vi "Get_Latest_Experiment_Settings.vi"(8 "error in (no error)":errorcluster) -> (0 "error out":errorcluster, 1 "Experiment":string[](array[string]), 2 "Group":string, 3 "Integer Timestamp":dbl)   [LabVIEW 2013]
uses:
  <vilib>/addons/database/Connection.llb/Conn Execute.vi
  <vilib>/addons/database/Recordset.llb/Rec Fetch Recordset Data (R).vi
  <vilib>/addons/database/Recordset.llb/Rec Destroy - Connection.vi
  <vilib>/addons/database/_DB Variant To Data/Database Variant To Data.xnode
  <vilib>/addons/database/NI_Database_API.lvlib
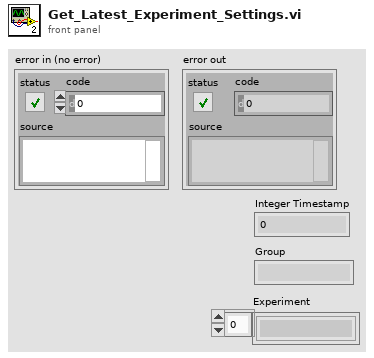
[diagram p1: front panel]
types:
  T1 = typedef "NI_Database_API.lvlib/Conn ObjectReference.ctl" = refnum<k1>
  T2 = typedef "NI_Database_API.lvlib/Rec ObjectReference.ctl" = refnum<k1>
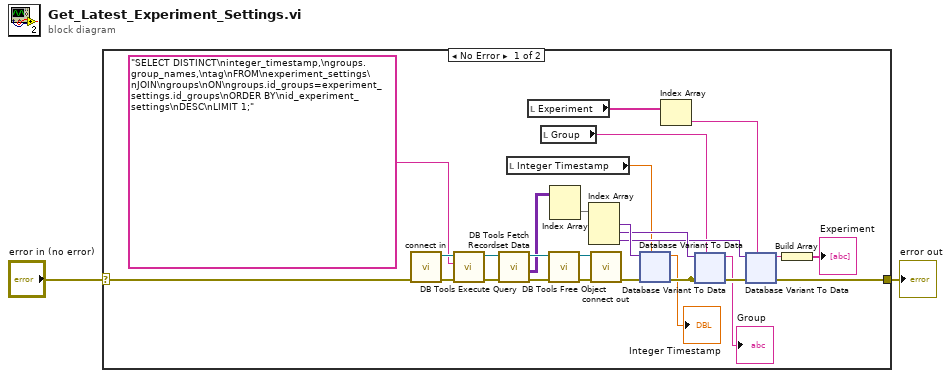
[diagram p0: block diagram]
diagram:
  n1 = case shown="No Error" "error in (no error)" {
    selector: "error in (no error)" -> [w4 w125]
    tunnel: [w16 w125] -> w1
    frame No Error {
      n2 = call "connect in.vi"("error in (no error)"=w4) -> ("error out"=w27:errorcluster, "Database Connection"=w26:T1)  [unwired: 6 in, 1 out]
      n3 = call-poly <vilib>:"DB Tools Execute Query.vi"("error in (no error)"=w27, "SQL query"="SELECT DISTINCT\ninteger_timestamp,\ngroups.group_names,\ntag\nFROM\nexperiment_settings\nJOIN\ngroups\nON\ngroups.id_groups=experiment_settings.id_groups\nORDER BY\nid_experiment_settings\nDESC\nLIMIT 1;" ("format string"), "connection reference"=w26) -> ("error out"=w25:errorcluster, "recordset reference"=w24:T2)  [unwired: 5 in]
      n4 = call-poly <vilib>:"DB Tools Fetch Recordset Data.vi"("error in (no error)"=w25, "recordset reference"=w24) -> ("error out"=w23:errorcluster, "recordset data"=w19:variant[][], "recordset reference out"=w28:T2)  [unwired: 3 in]
      n5 = local read "Integer Timestamp"() -> (w12:dbl)
      n6 = local read "Experiment"() -> (w10:string[])
      n7 = local read "Group"() -> (w11:string)
      n8 = call-poly <vilib>:"DB Tools Free Object.vi"("error in (no error)"=w23, "recordset reference"=w28) -> ("error out"=w21:errorcluster, "connection reference"=w22:T1)  [unwired: 8 in]
      n9 = Index Array(array=w19) -> (element=w18:variant[])  [unwired: 2 in]
      n10 = Index Array(array=w18) -> (element #1=w17:variant, element #2=w14:variant, element #3=w13:variant)  [unwired: 3 in]
      n11 = call "connect out.vi"("error in (no error)"=w21, "connection reference"=w22) -> ("error out"=w20:errorcluster)  [unwired: 9 in]
      n12 = xnode "Database Variant To Data"("database variant"=w17, "error in (no error)"=w20, "type"=w12) -> ("data"=→"Integer Timestamp":dbl, "error out"=w16:errorcluster)
      n13 = Index Array(array=w10) -> (element=w9:string)  [unwired: 1 in]
      n14 = xnode "Database Variant To Data"("database variant"=w14, "error in (no error)"=w16, "type"=w11) -> ("data"=→"Group":string, "error out"=w15:errorcluster)
      n15 = xnode "Database Variant To Data"("database variant"=w13, "error in (no error)"=w15, "type"=w9) -> ("data"=w6:string)  [unwired: 1 out]
      n16 = Build Array(w6) -> (→"Experiment":string[])
    }
    frame Error {
    }
  }
  "error out" <- w1
